vi "Read Ini File Instrument.vi"(8 "error in (no error)":errorcluster, 10 "Escala":string, 11 "Refnum in":T2) -> (0 "error out":errorcluster, 2 "Ini Output":T1, 3 "Refnum out":T2)   [LabVIEW 2015]
uses:
  <vilib>/Utility/config.llb/Config Data RefNum.ctl
  controls/Ini File Output.ctl
  <vilib>/Utility/config.llb/Read Key (String).vi
  <vilib>/Utility/config.llb/Read Key (Double).vi
  <vilib>/Utility/config.llb/Read Key (I32).vi
  <vilib>/Utility/config.llb/Read Key (Boolean).vi
  <vilib>/Utility/config.llb/NI_LVConfig.lvlib
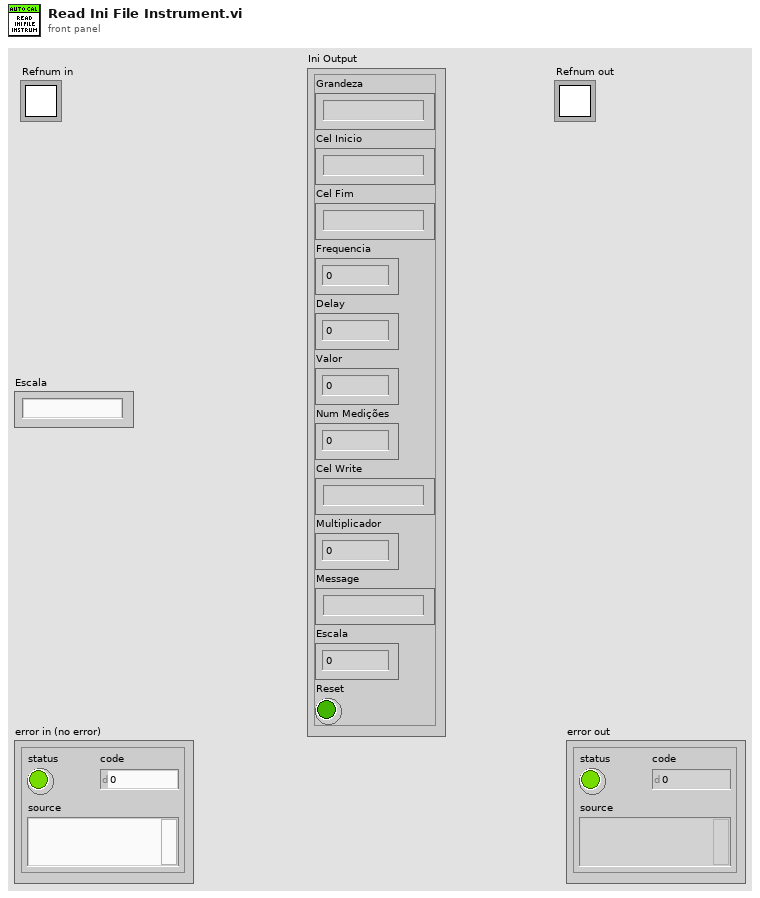
[diagram p1: front panel]
types:
  T1 = typedef "Ini File Output.ctl" = cluster{"Grandeza":string, "Cel Inicio":string, "Cel Fim":string, "Frequencia":dbl, "Delay":dbl, "Valor":dbl, "Num Medições":i32, "Cel Write":string, "Multiplicador":dbl, "Message":string, "Escala":dbl, "Reset":bool}
  T2 = typedef "NI_LVConfig.lvlib/Config Data RefNum.ctl" = refnum<k1>
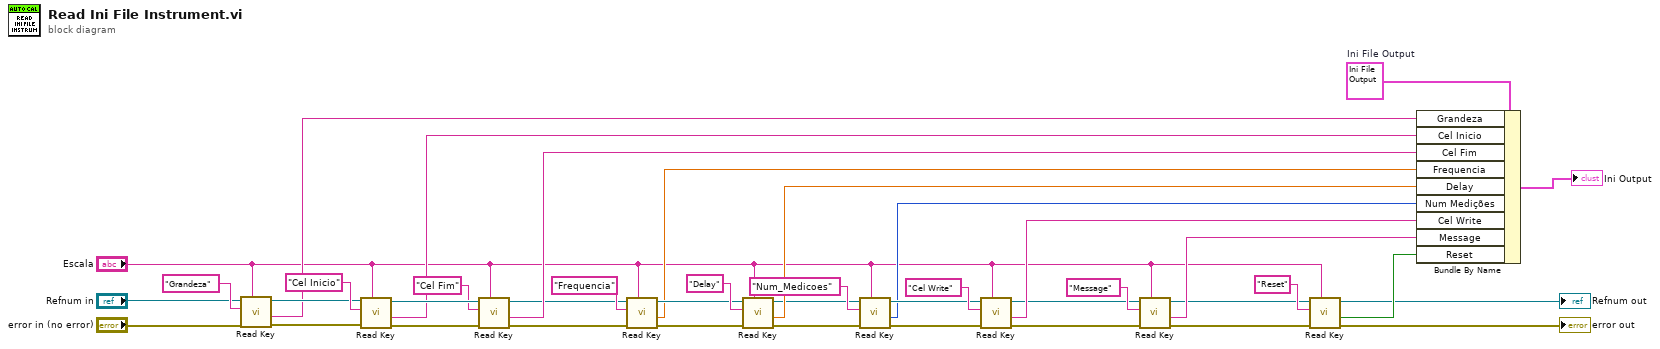
[diagram p0: block diagram]
diagram:
  w32 = T1 {"Grandeza"="", "Cel Inicio"="", "Cel Fim"="", "Frequencia"=0.0, "Delay"=0.0, "Valor"=0.0, "Num Medições"=0, "Cel Write"="", "Multiplicador"=0.0, "Message"="", "Escala"=0.0, "Reset"=FALSE}  # Ini File Output
  n1 = call-poly <vilib>:"Read Key.vi"("section"="Escala", "error in (no error)"="error in (no error)", "key"="Grandeza", "refnum"="Refnum in") -> ("error out"=w33:errorcluster, "value"=w31:string, "refnum out"=w34:T2)  [unwired: 4 in, 1 out]
  n2 = call-poly <vilib>:"Read Key.vi"("section"="Escala", "error in (no error)"=w33, "key"="Cel Inicio", "refnum"=w34) -> ("error out"=w41:errorcluster, "value"=w30:string, "refnum out"=w40:T2)  [unwired: 4 in, 1 out]
  n3 = call-poly <vilib>:"Read Key.vi"("section"="Escala", "error in (no error)"=w41, "key"="Cel Fim", "refnum"=w40) -> ("error out"=w25:errorcluster, "value"=w29:string, "refnum out"=w26:T2)  [unwired: 4 in, 1 out]
  n4 = call-poly <vilib>:"Read Key.vi"("section"="Escala", "error in (no error)"=w25, "key"="Frequencia", "refnum"=w26) -> ("error out"=w23:errorcluster, "value"=w22:dbl, "refnum out"=w24:T2)  [unwired: 4 in, 1 out]
  n5 = call-poly <vilib>:"Read Key.vi"("section"="Escala", "error in (no error)"=w23, "key"="Delay", "refnum"=w24) -> ("error out"=w16:errorcluster, "value"=w21:dbl, "refnum out"=w17:T2)  [unwired: 4 in, 1 out]
  n6 = call-poly <vilib>:"Read Key.vi"("section"="Escala", "error in (no error)"=w16, "key"="Num_Medicoes", "refnum"=w17) -> ("error out"=w14:errorcluster, "value"=w12:i32, "refnum out"=w15:T2)  [unwired: 4 in, 1 out]
  n7 = call-poly <vilib>:"Read Key.vi"("section"="Escala", "error in (no error)"=w14, "key"="Cel Write", "refnum"=w15) -> ("error out"=w9:errorcluster, "value"=w13:string, "refnum out"=w10:T2)  [unwired: 4 in, 1 out]
  n8 = call-poly <vilib>:"Read Key.vi"("section"="Escala", "error in (no error)"=w9, "key"="Message", "refnum"=w10) -> ("error out"=w5:errorcluster, "value"=w8:string, "refnum out"=w6:T2)  [unwired: 4 in, 1 out]
  n9 = call-poly <vilib>:"Read Key.vi"("section"="Escala", "error in (no error)"=w5, "key"="Reset", "refnum"=w6) -> ("error out"=→"error out":errorcluster, "value"=w3:bool, "refnum out"=→"Refnum out":T2)  [unwired: 4 in, 1 out]
  n10 = Bundle By Name(cluster=w32, "Grandeza"=w31, "Cel Inicio"=w30, "Cel Fim"=w29, "Frequencia"=w22, "Delay"=w21, "Num Medições"=w12, "Cel Write"=w13, "Message"=w8, "Reset"=w3) -> (→"Ini Output":T1)
